vi "InitFromCfgFile.vi"(8 "error in (no error)":errorcluster, 10 "configuration file path":path, 11 "ByteGSAPIBase in":refnum<class "ByteGSAPIBase.lvclass">) -> (0 "error out":errorcluster, 3 "ByteGSAPIBase out":refnum<class "ByteGSAPIBase.lvclass">)   [LabVIEW 2019, in "ByteGSWebAPI.lvlib" / "ByteGSAPIBase.lvclass"]
uses:
  ByteGSAPIBase.lvclass
  <vilib>/Bytelabs/ByteREST/CfgLoaders/LoaderBase/ServerParams.ctl
  <vilib>/Bytelabs/ByteREST/ByteRESTClass/ByteRESTBase/Auth/Authentication_type.ctl
  <vilib>/Bytelabs/ByteREST/ByteRESTClass/ByteRESTBase/RESTBase.lvclass
  <vilib>/Bytelabs/ByteREST/CfgLoaders/LoaderConstant/RESTLoaderConstant.lvclass/RESTLoaderConstant.ctl
  ByteGSAPIBase.lvclass/ByteGSAPIBase.ctl
  <vilib>/Bytelabs/ByteREST/CfgLoaders/LoaderConstant/RESTLoaderConstant.lvclass
  C:/Program Files (x86)/National Instruments/LabVIEW 2019/vi.lib/Bytelabs/ByteREST/CfgLoaders/LoaderBase/RESTLoaderBase.lvclass
  <vilib>/Utility/config.llb/Read Key (U32).vi
  <vilib>/Utility/config.llb/Read Key (String).vi
  <vilib>/Utility/config.llb/NI_LVConfig.lvlib
  <vilib>/Bytelabs/ByteREST/CfgLoaders/LoaderBase/RESTLoaderBase.lvclass
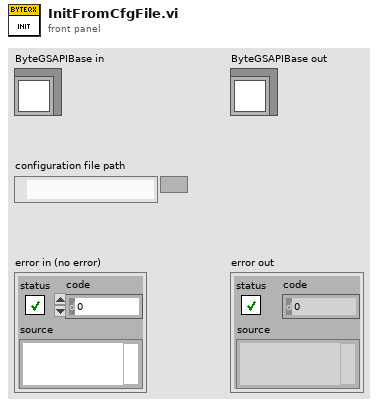
[diagram p1: front panel]
types:
  T1 = typedef "ByteREST.lvlib/RESTLoaderBase.lvclass/ServerParams.ctl" = cluster{"API Root":string, "verify server":bool, "Version (no version)":string, "Port (protocol specific)":u16, "Base URL":string, "Auth type":T2, "Auth string":string, "timeout (10000)":i32, "Token preamble (Token)":string, "Token empty preamble (False)":bool, "Token header key (Authorization)":string}
  T2 = typedef "ByteREST.lvlib/RESTBase.lvclass/Authentication_type.ctl" = enum16{"Token"}
  T3 = typedef "NI_LVConfig.lvlib/Config Data RefNum.ctl" = refnum<k1>
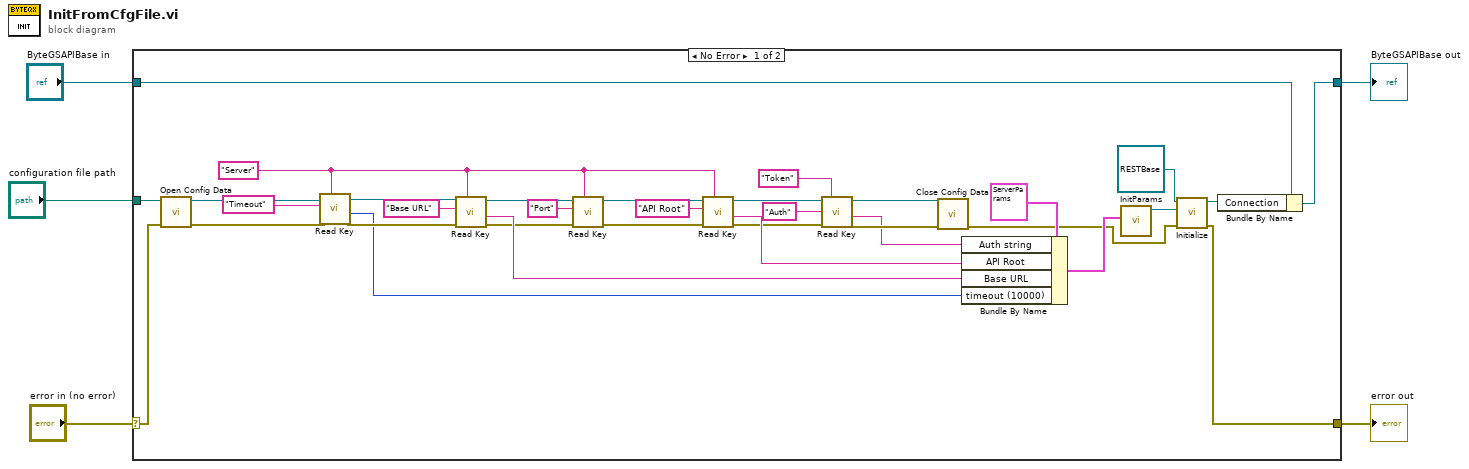
[diagram p0: block diagram]
diagram:
  n1 = case shown="No Error" "error in (no error)" {
    selector: "error in (no error)" -> [w27 w41]
    tunnel: [w28 w41] -> w4
    tunnel: [w36 w40] -> w2
    tunnel: "ByteGSAPIBase in" -> [w32 w40]
    tunnel: "configuration file path" -> [w37 _]
    frame No Error {
      w15 = "Server" ("section")
      n2 = call <vilib>:"Open Config Data.vi"("error in (no error)"=w27, "configuration file path"=w37) -> ("error out"=w39:errorcluster, "refnum"=w38:T3)  [unwired: 7 in, 1 out]
      n3 = call-poly <vilib>:"Read Key.vi"("section"=w15, "error in (no error)"=w39, "key"="Timeout", "refnum"=w38) -> ("error out"=w24:errorcluster, "value"=w22:u32, "refnum out"=w25:T3)  [unwired: 4 in, 1 out]
      n4 = call-poly <vilib>:"Read Key.vi"("section"=w15, "error in (no error)"=w24, "key"="Base URL", "refnum"=w25) -> ("error out"=w20:errorcluster, "value"=w21:string, "refnum out"=w19:T3)  [unwired: 4 in, 1 out]
      n5 = call-poly <vilib>:"Read Key.vi"("section"=w15, "error in (no error)"=w20, "key"="Port", "refnum"=w19) -> ("error out"=w16:errorcluster, "refnum out"=w17:T3)  [unwired: 4 in, 2 out]
      n6 = call-poly <vilib>:"Read Key.vi"("section"=w15, "error in (no error)"=w16, "key"="API Root", "refnum"=w17) -> ("error out"=w11:errorcluster, "value"=w13:string, "refnum out"=w10:T3)  [unwired: 4 in, 1 out]
      n7 = call-poly <vilib>:"Read Key.vi"("section"="Token", "error in (no error)"=w11, "key"="Auth", "refnum"=w10) -> ("error out"=w8:errorcluster, "value"=w6:string, "refnum out"=w9:T3)  [unwired: 4 in, 1 out]
      n8 = call <vilib>:"Close Config Data.vi"("error in (no error)"=w8, "refnum"=w9) -> ("error out"=w26:errorcluster)  [unwired: 8 in, 1 out]
      n9 = Bundle By Name(cluster=T1 {"API Root"="", "verify server"=FALSE, "Version (no version)"="", "Port (protocol specific)"=0, "Base URL"="", "Auth type"=enum."Token", "Auth string"="", "timeout (10000)"=10000, "Token preamble (Token)"="", "Token empty preamble (False)"=FALSE, "Token header key (Authorization)"=""} ("Cluster"), "Auth string"=w6, "API Root"=w13, "Base URL"=w21, "timeout (10000)"=w22) -> (w35:T1)
      n10 = call <vilib>:"InitParams.vi"("Cluster"=w35) -> ("RESTLoaderConstant out"=w33:refnum<class "RESTLoaderConstant.lvclass">)  [unwired: 10 in]
      n11 = call-dynamic "Initialize.vi"("error in (no error)"=w26, "RESTLoader"=w33, "REST in"=refnum<class "RESTBase.lvclass"> refnum) -> ("error out"=w28:errorcluster, "REST out"=w30:refnum<class "RESTBase.lvclass">)  [unwired: 7 in]
      n12 = Bundle By Name(cluster=w32, "Connection"=w30) -> (w36:refnum<class "ByteGSAPIBase.lvclass">)
    }
    frame Error {
    }
  }
  "error out" <- w4
  "ByteGSAPIBase out" <- w2
